vi "Température to puissance.vi"(10 "Longueur d'onde":dbl, 11 "Température max":dbl) -> (3 "Puissance":dbl)   [LabVIEW 2018]
uses:
  <vilib>/imath/engines/lvmath2/RunTimeEngine/Managers/WorkSpace/UID Generator.vi
  <vilib>/imath/engines/lvmath2/RunTimeEngine/RunTimeType/NIMS_RunTimeType_From StrictType (excl LVString).vi
  <instcachedir>/0/NIMS_RunTimeType_From StrictType (excl LVString)_E7E34A65C99947108168652BAD14964D.lvgen/NIMS_RunTimeType_From StrictType (excl LVString)_E7E34A65C99947108168652BAD14964D_000.vi
  <vilib>/imath/engines/lvmath2/RunTimeEngine/LocalVariableDefStatement/MC_LocalVariableDefStatement_Display.vi
  <vilib>/imath/engines/lvmath2/RunTimeEngine/Managers/SymbolTable/Clear UID.vi
  <vilib>/imath/engines/lvmath2/RunTimeEngine/NodeEndStatement/NIMS_NodeEndStatement_Output.vi
  <instcachedir>/0/NIMS_NodeEndStatement_Output_53EC0D466D134D7ABD903AC30B43404B.lvgen/NIMS_NodeEndStatement_Output_53EC0D466D134D7ABD903AC30B43404B_001.vi
  <vilib>/imath/engines/lvmath2/RunTimeEngine/ErrorHandling/NIMS_Finalize Error.vi
  <vilib>/imath/engines/lvmath2/RunTimeEngine/Managers/SymbolTable/NIMS_WorkSpace.lvlib
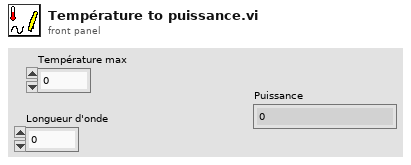
[diagram p1: front panel]
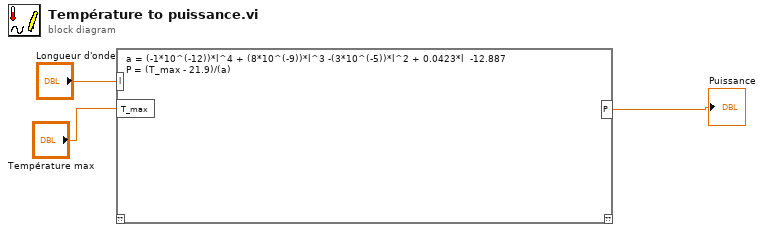
[diagram p0: block diagram]
diagram:
  n1 = mathscript code="a = (-1*10^(-12))*l^4 + (8*10^(-9))*l^3 -(3*10^(-5))*l^2 + 0.0423*l  -12.887\nP = (T_max - 21.9)/(a)"("l"="Longueur d'onde", "T_max"="Température max") -> ("P"=→"Puissance":dbl)  [unwired: 1 in, 1 out]
